vi "Read Section.vi"(8 "error in (no error)":errorcluster, 9 "Data In":variant, 10 "Section Name":string, 11 "Configuration File in":refnum<class "Configuration File.lvclass">) -> (0 "error out":errorcluster, 1 "Found section and keys?":bool, 2 "Data Out":variant, 3 "Configuration File out":refnum<class "Configuration File.lvclass">)   [LabVIEW 2019, in "Configuration File.lvlib" / "Configuration File.lvclass"]
doc: "This VI reads a section of the configuration file and returns a variant with all the keys as its attributes.\n\nYou can wire a Data In to load the new configuration to a previouly read one. This will replace the existing keys and create a new ones, but not delete those which exit and were not read."
uses:
  Configuration File.lvclass
  Configuration File.lvclass/Configuration File.ctl
  <vilib>/Utility/config.llb/Read Key (Boolean).vi
  <vilib>/Utility/config.llb/Read Key (U32).vi
  <vilib>/Utility/config.llb/Read Key (I32).vi
  <vilib>/Utility/config.llb/Read Key (Path).vi
  <vilib>/Utility/config.llb/Read Key (Double).vi
  <vilib>/Utility/config.llb/Read Key (String).vi
  <vilib>/Utility/config.llb/NI_LVConfig.lvlib
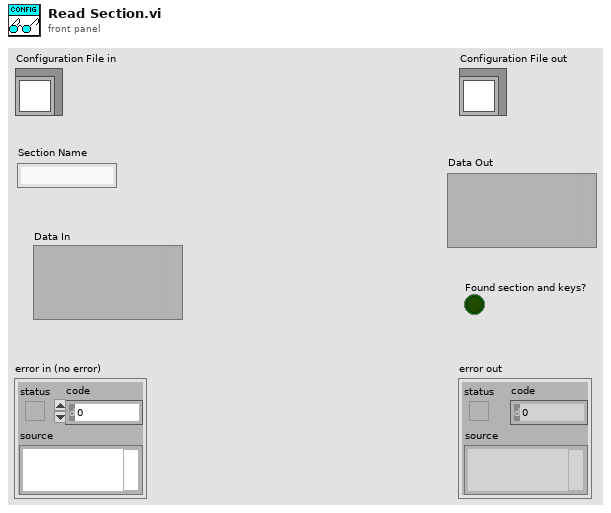
[diagram p1: front panel]
types:
  T1 = typedef "NI_LVConfig.lvlib/Config Data RefNum.ctl" = refnum<k1>
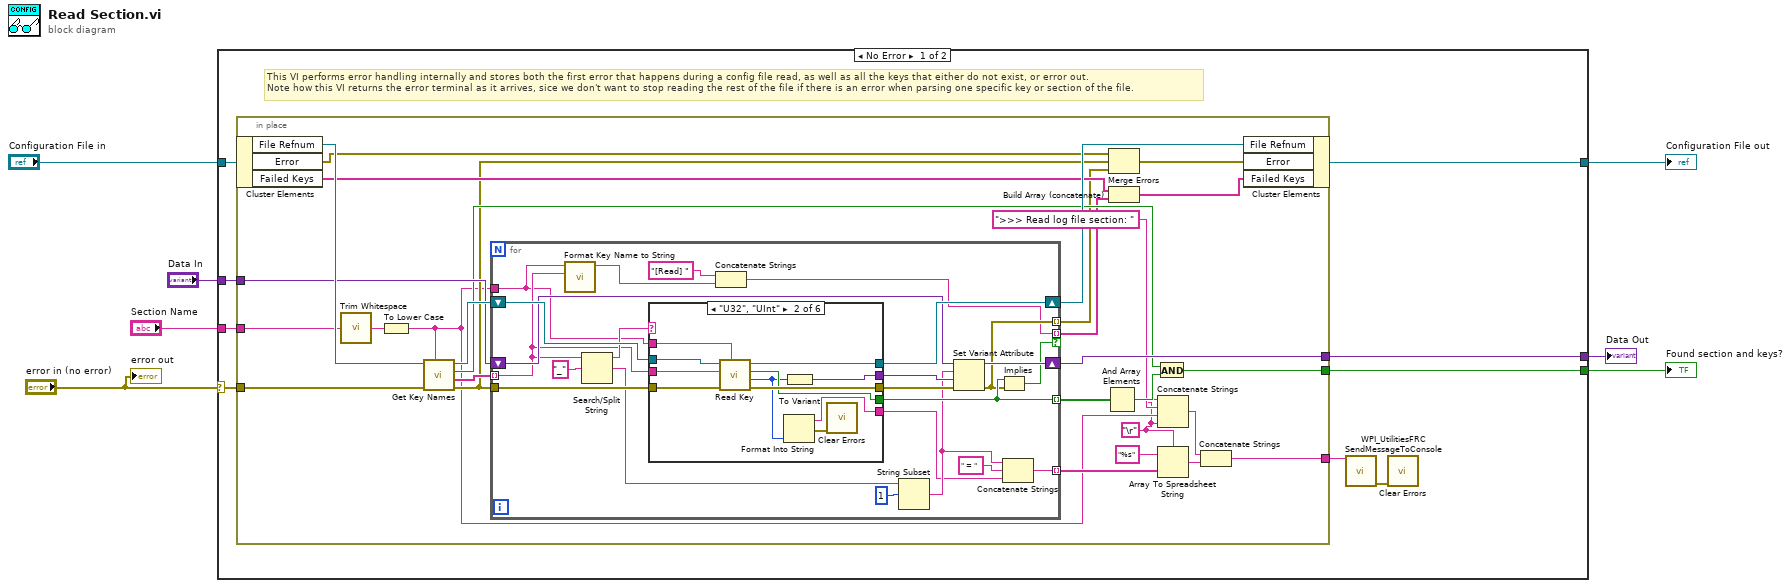
[diagram p0: block diagram]
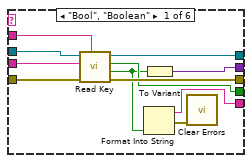
[diagram p2: hidden frame]
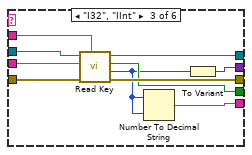
[diagram p3: hidden frame]
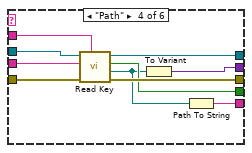
[diagram p4: hidden frame]
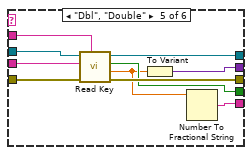
[diagram p5: hidden frame]
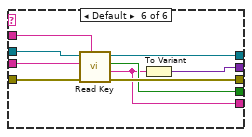
[diagram p6: hidden frame]
diagram:
  n1 = case shown="No Error" "error in (no error)" {
    selector: "error in (no error)" -> [w10 _]
    tunnel: [w14 w130] -> w6
    tunnel: "Configuration File in" -> [w13 w130]
    tunnel: [w16 w129] -> w5
    tunnel: "Section Name" -> [w15 _]
    tunnel: "Data In" -> [w12 w129]
    tunnel: [w11 _] -> w2
    frame No Error {
      # "This VI performs error handling internally and stores both the first error that happens during a config file read, as well as all the keys that either do not exist, or error out. \nNote how this VI returns the error terminal as it arrives, sice we don't want to stop reading the rest of the file if there is an error when parsing one specific key or section of the file."
      n2 = in-place {
        in-place-border: w10 -> [w43]
        in-place-border: [w39] -> w16
        in-place-border: w12 -> [w38]
        in-place-border: [w33] -> w11
        in-place-border: w15 -> [w35]
        in-place-border: [w18] -> w9
        w17 = "\r"
        n3 = in-place-cluster #1(w13) -> ("File Refnum"=w44:T1, "Error"=w27:errorcluster, "Failed Keys"=w31:string[])
        n4 = call <vilib>:"Trim Whitespace.vi"("string"=w35) -> ("trimmed string"=w36:string)  [unwired: 1 in]
        n5 = To Lower Case(string=w36) -> (all lower case string=w19:string)
        n6 = call <vilib>:"Get Key Names.vi"("section"=w19, "error in (no error)"=w43, "refnum"=w44) -> ("error out"=w26:errorcluster, "key names"=w42:string[], "section exists?"=w32:bool, "refnum out"=w40:T1)  [unwired: 5 in]
        n7 = for {
          tunnel: w42 -> [w56] mode=indexing
          shift-right: [w63] -> w41
          shift-left: w40 -> [w64]
          tunnel: w19 -> [w55]
          shift-right: [w61] -> w39
          shift-left: w38 -> [w62]
          tunnel: [w53] -> w37 mode=indexing
          tunnel: [w46] -> w29 mode=indexing if=w52
          tunnel: w26 -> [w67]
          tunnel: [w51] -> w25 mode=indexing
          tunnel: [w47] -> w24 mode=indexing
          n8 = call "Format Key Name to String.vi"("Key"=w56, "Section"=w55) -> ("String out"=w54:string)  [unwired: 9 in]
          n9 = Search/Split String(string=w56, search string/char (-)="_") -> (substring before match=w57:string, match + rest of string=w58:string)  [unwired: 1 in, 1 out]
          n10 = case shown="\"U32\", \"UInt\"" w57 {
            tunnel: w67 -> [w78 w89 w99 w109 w119 w128]
            tunnel: [w77 w88 w98 w108 w118 w127] -> w65
            tunnel: w64 -> [w76 w87 w97 w107 w117 w126]
            tunnel: [w75 w86 w96 w106 w116 w125] -> w63
            tunnel: w56 -> [w74 w85 w95 w105 w115 w124]
            tunnel: w55 -> [w73 w84 w94 w104 w114 w123]
            tunnel: [w72 w83 w93 w103 w113 w122] -> w59
            tunnel: [w71 w82 w92 w102 w112 w121] -> w53
            tunnel: [w69 w79 w91 w100 w111 w120] -> w48
            frame "Bool", "Boolean" {
              n11 = call-poly <vilib>:"Read Key.vi"("section"=w73, "error in (no error)"=w78, "key"=w74, "refnum"=w76) -> ("error out"=w77:errorcluster, "value"=w70:bool, "found?"=w71:bool, "refnum out"=w75:T1)  [unwired: 4 in]
              n12 = Format Into String(w70) -> (resulting string=w69:string, error out=w68:errorcluster)  [unwired: 3 in]
              n13 = To Variant(anything=w70) -> (Variant=w72:variant)
              n14 = call <vilib>:"Clear Errors.vi"("error in (no error)"=w68) -> ()  [unwired: 5 in, 2 out]
            }
            frame "U32", "UInt" {
              n15 = call-poly <vilib>:"Read Key.vi"("section"=w84, "error in (no error)"=w89, "key"=w85, "refnum"=w87) -> ("error out"=w88:errorcluster, "value"=w80:u32, "found?"=w82:bool, "refnum out"=w86:T1)  [unwired: 4 in]
              n16 = Format Into String(w80) -> (resulting string=w79:string, error out=w81:errorcluster)  [unwired: 3 in]
              n17 = To Variant(anything=w80) -> (Variant=w83:variant)
              n18 = call <vilib>:"Clear Errors.vi"("error in (no error)"=w81) -> ()  [unwired: 5 in, 2 out]
            }
            frame "I32", "IInt" {
              n19 = call-poly <vilib>:"Read Key.vi"("section"=w94, "error in (no error)"=w99, "key"=w95, "refnum"=w97) -> ("error out"=w98:errorcluster, "value"=w90:i32, "found?"=w92:bool, "refnum out"=w96:T1)  [unwired: 4 in]
              n20 = Number To Decimal String(number=w90, width (-)=w90) -> (decimal integer string=w91:string)
              n21 = To Variant(anything=w90) -> (Variant=w93:variant)
            }
            frame "Path" {
              n22 = call-poly <vilib>:"Read Key.vi"("section"=w104, "error in (no error)"=w109, "key"=w105, "refnum"=w107) -> ("error out"=w108:errorcluster, "value"=w101:path, "found?"=w102:bool, "refnum out"=w106:T1)  [unwired: 4 in]
              n23 = To Variant(anything=w101) -> (Variant=w103:variant)
              n24 = Path To String(path=w101) -> (string=w100:string)
            }
            frame "Dbl", "Double" {
              n25 = call-poly <vilib>:"Read Key.vi"("section"=w114, "error in (no error)"=w119, "key"=w115, "refnum"=w117) -> ("error out"=w118:errorcluster, "value"=w110:dbl, "found?"=w112:bool, "refnum out"=w116:T1)  [unwired: 4 in]
              n26 = To Variant(anything=w110) -> (Variant=w113:variant)
              n27 = Number To Fractional String(number=w110) -> (F-format string=w111:string)  [unwired: 3 in]
            }
            frame Default {
              n28 = call-poly <vilib>:"Read Key.vi"("section"=w123, "error in (no error)"=w128, "key"=w124, "refnum"=w126) -> ("error out"=w127:errorcluster, "value"=w120:string, "found?"=w121:bool, "refnum out"=w125:T1)  [unwired: 4 in]
              n29 = To Variant(anything=w120) -> (Variant=w122:variant)
            }
          }
          n30 = Concatenate Strings("[Read] " ("string"), w54) -> (w46:string)
          n31 = String Subset(string=w58, offset (0)=1) -> (substring=w50:string)  [unwired: 1 in]
          n32 = Set Variant Attribute(Variant=w62, name=w50, value=w59, error in=w65) -> (Variant out=w61:variant, error out=w51:errorcluster)  [unwired: 1 out]
          n33 = Implies(1:w51, 2:w53) -> (0:w52:bool)
          n34 = Concatenate Strings(w50, " = " ("string"), w48) -> (w47:string)
        }
        n35 = And Array Elements(Boolean array=w37) -> (logical AND=w34:bool)
        n36 = Merge Errors(w27, w26, w25) -> (w28:errorcluster)
        n37 = Build Array (concatenate)(w31, w29) -> (w30:string[])
        n38 = And(x=w32, y=w34) -> (x .and. y?=w33:bool)
        n39 = Concatenate Strings(w17, ">>> Read log file section: " ("string"), w19, w17) -> (w21:string)
        n40 = Array To Spreadsheet String(delimiter (Tab)=w17, array=w24, 3:"%s" ("format string")) -> (spreadsheet string=w22:string)
        n41 = Concatenate Strings(w21, w22) -> (w18:string)
        n42 = in-place-cluster #1("File Refnum"=w41, "Error"=w28, "Failed Keys"=w30) -> (w14:refnum<class "Configuration File.lvclass">)
      }
      n43 = call <vilib>:"WPI_UtilitiesFRC SendMessageToConsole.vi"("Message"=w9) -> ("error out"=w8:errorcluster)  [unwired: 14 in]
      n44 = call <vilib>:"Clear Errors.vi"("error in (no error)"=w8) -> ()  [unwired: 5 in, 2 out]
    }
    frame Error {
    }
  }
  "Configuration File out" <- w6
  "Data Out" <- w5
  "Found section and keys?" <- w2
  "error out" <- "error in (no error)"
